vi "TCP_SenData.vi"(8 "error in":errorcluster, 10 "Server":T1 {"Knob" scale=0.0..10.0; "Horizontal Fill Slide" scale=0.0..10.0}, 11 "Clients":refnum<k5>[](array[refnum])) -> (0 "error out":errorcluster, 1 "Current Data":dbl, 2 "# of Connections":i32, 3 "Clients":refnum<k5>[](array[refnum]), 5 "concatenated string":string)   [LabVIEW 2020, in "TCP_Server.lvlib"]
uses:
  TCP_Server.lvlib
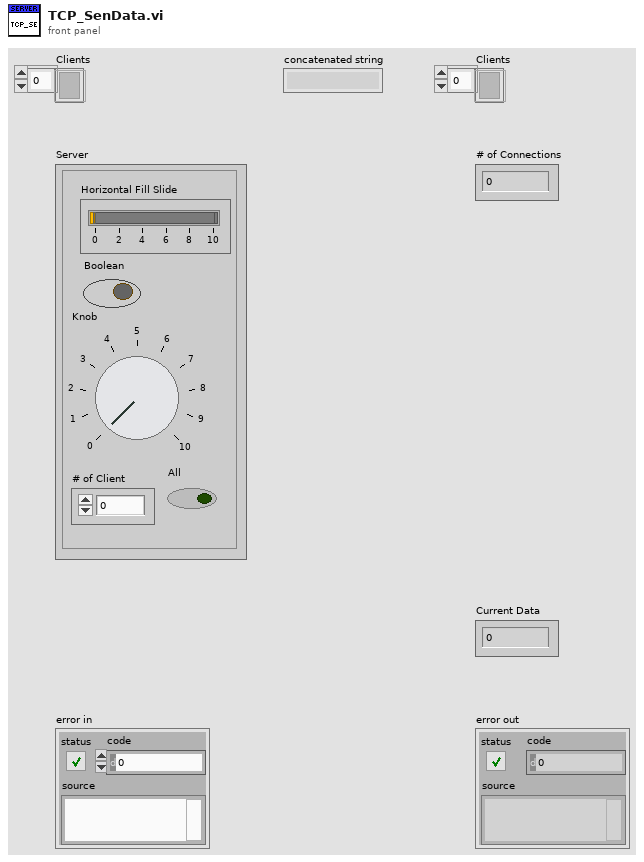
[diagram p1: front panel]
types:
  T1 = cluster{"Horizontal Fill Slide":dbl, "Knob":dbl, "Boolean":bool, "# of Client":i32, "All":bool}
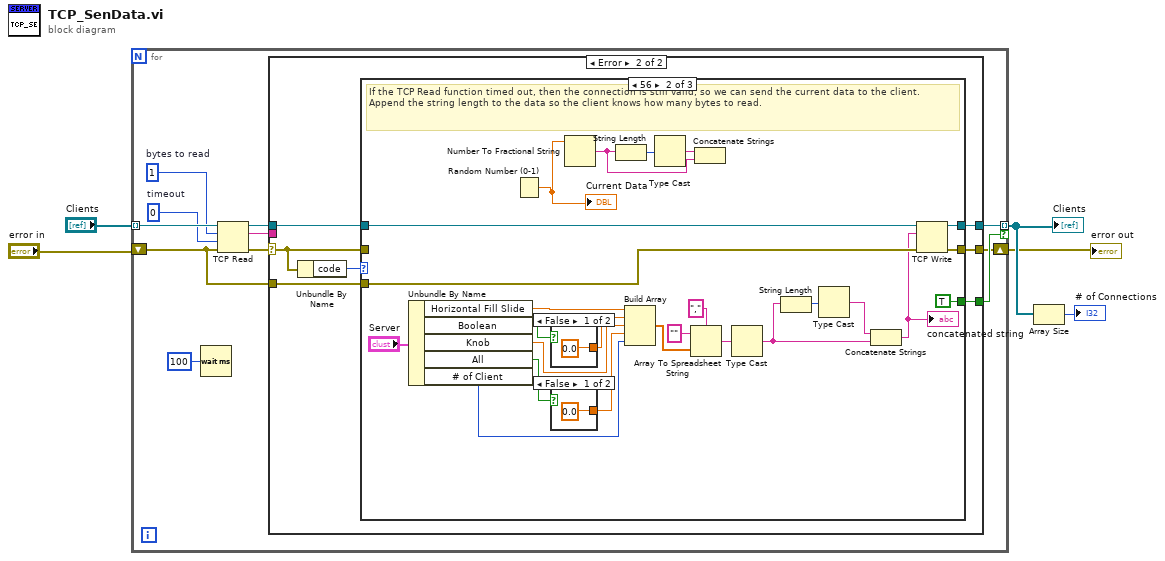
[diagram p0: block diagram]
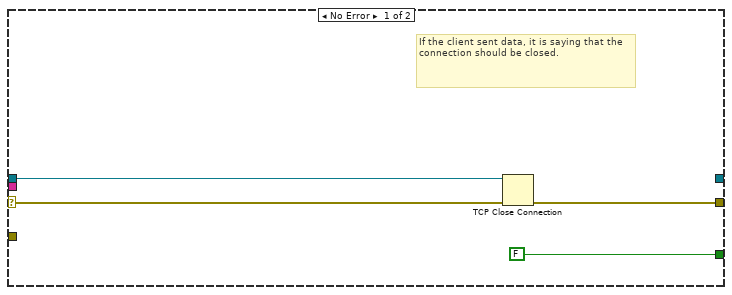
[diagram p2: hidden frame]
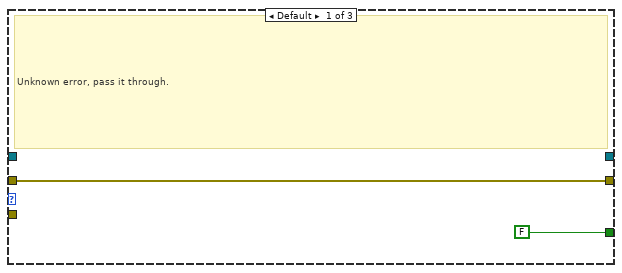
[diagram p3: hidden frame]
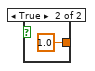
[diagram p4: hidden frame]
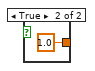
[diagram p5: hidden frame]
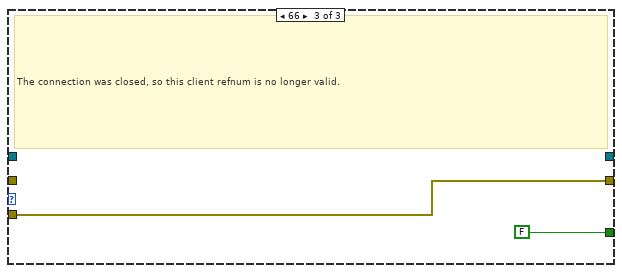
[diagram p6: hidden frame]
diagram:
  n1 = for {
    tunnel: "Clients" -> [w16] mode=indexing
    shift-right: [w8] -> w1
    shift-left: "error in" -> [w7]
    tunnel: [w10] -> w4 mode=indexing if=w9
    w13 = 0  # timeout
    w14 = 1  # bytes to read
    n2 = Wait (ms)(milliseconds to wait=u32 100) -> ()  [unwired: 1 out]
    n3 = TCP Read(connection ID=w16, bytes to read=w14, error in (no error)=w7, 9:w13) -> (connection ID out=w15:refnum<k5>, data out=w11:string, error out=w12:errorcluster)  [unwired: 1 out]
    n4 = case shown="Error" w12 {
      selector: w12 -> [w19 w26]
      tunnel: w15 -> [w20 w23]
      tunnel: w11 -> [_ _]
      tunnel: [_ w21] -> w10
      tunnel: [FALSE w22] -> w9
      tunnel: [w17 w25] -> w8
      tunnel: w7 -> [_ w24]
      frame No Error {
        # "If the client sent data, it is saying that the connection should be closed."
        # "If the client sent data, it is saying that the connection should be closed."
        n5 = TCP Close Connection(connection ID=w20, error in (no error)=w19) -> (error out=w17:errorcluster)  [unwired: 2 out]
      }
      frame Error {
        # "Ignore connection closed and timeout errors"
        n6 = Unbundle By Name(w26) -> ("code"=w27:i32)
        n7 = case shown="56" w27 {
          tunnel: w26 -> [w29 _ _]
          tunnel: [w29 w54 w60] -> w25
          tunnel: w24 -> [_ w50 w60]
          tunnel: w23 -> [_ w53 _]
          tunnel: [FALSE TRUE FALSE] -> w22
          tunnel: [_ w52 _] -> w21
          frame Default {
            # "Unknown error, pass it through."
          }
          frame 56 {
            # "If the TCP Read function timed out, then the connection is still valid, so we can send the current data to the client. Append the string length to the data so the client knows how many bytes to read."
            n8 = Unbundle By Name("Server") -> ("Horizontal Fill Slide"=w42:dbl, "Boolean"=w48:bool, "Knob"=w46:dbl, "All"=w32:bool, "# of Client"=w30:i32)
            n9 = Random Number (0-1)() -> (number: 0 to 1=w35:dbl)
            "Current Data" <- w35
            n10 = case shown="False" w48 {
              tunnel: [0.0 1.0] -> w49
              frame False {
              }
              frame True {
              }
            }
            n11 = case shown="False" w32 {
              tunnel: [0.0 1.0] -> w31
              frame False {
              }
              frame True {
              }
            }
            n12 = Number To Fractional String(number=w35) -> (F-format string=w36:string)  [unwired: 3 in]
            n13 = String Length(string=w36) -> (length=w37:i32)
            n14 = Build Array(w42, w49, w46, w31, w30) -> (w47:dbl[])
            n15 = Type Cast(x=w37) -> (*(type *) &x=w38:string)  [unwired: 1 in]
            n16 = Array To Spreadsheet String(delimiter (Tab)=",", array=w47, 3:"" ("format string")) -> (spreadsheet string=w39:string)
            n17 = Concatenate Strings(w38, w36) -> ()  [unwired: 1 out]
            n18 = Type Cast(x=w39) -> (*(type *) &x=w40:string)  [unwired: 1 out]
            n19 = String Length(string=w40) -> (length=w45:i32)
            n20 = Type Cast(x=w45) -> (*(type *) &x=w41:string)  [unwired: 1 out]
            n21 = Concatenate Strings(w41, w40) -> (w34:string)
            "concatenated string" <- w34
            n22 = TCP Write(connection ID=w53, data in=w34, error in (no error)=w50) -> (connection ID out=w52:refnum<k5>, error out=w54:errorcluster)  [unwired: 2 out]
          }
          frame 66 {
            # "The connection was closed, so this client refnum is no longer valid."
          }
        }
      }
    }
  }
  "Clients" <- w4
  "error out" <- w1
  n23 = Array Size(array=w4) -> (size(s)=→"# of Connections":i32)
